vi "GUI_148_BeamPointingCams.vi"() -> ()   [LabVIEW 2013]
uses:
  Shared/GUI_Template/GUI_master/tcp_new_data_event.ctl
  Shared/GUI_Template/GUI_master/tcp new data cluster.ctl
  Control 2.ctl
  General GUIs/Device GUIs/GUI_Cameras/Controls/Crosshair type def.ctl
  <userlib>/_OpenG.lib/array/array.llb/Filter 1D Array with Scalar (String)__ogtk.vi
panel:
  in  "kHzMode":bool
  in  "DiodeMode":bool
  in  "Analysis::10":bool
  out "MeanCounts::10":dbl caption="updating?" min=0.0 max=999999999.0 format="%_4g"
  in  "Analysis::9":bool
  out "MeanCounts::9":dbl caption="updating?" min=0.0 max=999999999.0 format="%_4g"
  in  "Analysis::8":bool
  out "MeanCounts::8":dbl caption="updating?" min=0.0 max=999999999.0 format="%_4g"
  in  "Analysis::7":bool
  out "MeanCounts::7":dbl caption="updating?" min=0.0 max=999999999.0 format="%_4g"
  in  "Analysis::6":bool
  out "MeanCounts::6":dbl caption="updating?" min=0.0 max=999999999.0 format="%_4g"
  in  "Analysis::5":bool
  out "MeanCounts::5":dbl caption="updating?" min=0.0 max=999999999.0 format="%_4g"
  in  "Analysis::4":bool
  out "MeanCounts::4":dbl caption="updating?" min=0.0 max=999999999.0 format="%_4g"
  in  "Analysis::3":bool
  out "MeanCounts::3":dbl caption="updating?" min=0.0 max=999999999.0 format="%_4g"
  in  "Analysis::2":bool
  out "MeanCounts::2":dbl caption="updating?" min=0.0 max=999999999.0 format="%_4g"
  in  "Target.Y::10":dbl=45.0 caption="y" min=0.0 max=2000.0 format="%#_6f"
  in  "Target.X::10":dbl=47.0 caption="x" min=0.0 max=2000.0 format="%#_6f"
  in  "TargetSize.Y::10":dbl=45.0 caption="y" min=2.0 max=3000.0 format="%#_6f"
  in  "TargetSize.X::10":dbl=47.0 caption="x" min=2.0 max=3000.0 format="%#_6f"
  out "image::10":T1(plugin-control) caption="UC_BCaveIn"
  in  "GUIdevice 10":T2="UC_BCaveIn"
  in  "exposure::10":dbl=0.001 caption="exposure" min=10.0 max=1000000.0 format="%_4p"
  out "image::8":T1(plugin-control) caption="UC_Beamline_In"
  in  "GUIdevice 8":T2="UC_Beamline_In"
  in  "triggerdelay::10":dbl=0.001 caption="triggerdelay" min=10.0 max=1000000.0 format="%_4p"
  in  "triggerdelay::9":dbl=0.001 caption="triggerdelay" min=20.0 max=500000.0 format="%_4p"
  in  "triggerdelay::8":dbl=0.001 caption="triggerdelay" min=0.0 max=900000.0 format="%_4p"
  in  "trigger::10":bool caption="Trigger"
  in  "trigger::9":bool caption="Trigger"
  in  "trigger::8":bool caption="Trigger"
  in  "exposure::9":dbl=0.001 caption="exposure" min=0.0001 max=1.0 format="%_4p"
  in  "exposure::8":dbl=0.001 caption="exposure" min=0.0001 max=1.0 format="%_4p"
  in  "TargetSize.Y::9":dbl=45.0 caption="y" min=2.0 max=3000.0 format="%#_6f"
  in  "TargetSize.X::9":dbl=47.0 caption="x" min=2.0 max=3000.0 format="%#_6f"
  in  "TargetSize.Y::8":dbl=45.0 caption="y" min=2.0 max=3000.0 format="%#_6f"
  in  "TargetSize.X::8":dbl=47.0 caption="x" min=2.0 max=3000.0 format="%#_6f"
  in  "Target.Y::9":dbl=45.0 caption="y" min=0.0 max=2000.0 format="%#_6f"
  in  "Target.X::9":dbl=47.0 caption="x" min=0.0 max=2000.0 format="%#_6f"
  in  "Target.Y::8":dbl=45.0 caption="y" min=0.0 max=2000.0 format="%#_6f"
  in  "Target.X::8":dbl=47.0 caption="x" min=0.0 max=2000.0 format="%#_6f"
  out "image::9":T1(plugin-control) caption="UC_Beamline_Out"
  in  "GUIdevice 9":T2="UC_Beamline_Out"
  in  "Color Box":u32(colorbox)
  in  "TargetSize.Y::7":dbl=45.0 caption="y" min=2.0 max=3000.0 format="%#_6f"
  in  "TargetSize.X::7":dbl=47.0 caption="x" min=2.0 max=3000.0 format="%#_6f"
  in  "TargetSize.Y::6":dbl=45.0 caption="y" min=2.0 max=3000.0 format="%#_6f"
  in  "TargetSize.X::6":dbl=47.0 caption="x" min=2.0 max=3000.0 format="%#_6f"
  in  "TargetSize.Y::5":dbl=45.0 caption="y" min=2.0 max=3000.0 format="%#_6f"
  in  "TargetSize.X::5":dbl=47.0 caption="x" min=2.0 max=3000.0 format="%#_6f"
  in  "TargetSize.Y::4":dbl=45.0 caption="y" min=2.0 max=3000.0 format="%#_6f"
  in  "TargetSize.X::4":dbl=47.0 caption="x" min=2.0 max=3000.0 format="%#_6f"
  in  "TargetSize.Y::3":dbl=163.0 caption="y" min=2.0 max=3000.0 format="%#_6f"
  in  "TargetSize.X::3":dbl=152.0 caption="x" min=2.0 max=3000.0 format="%#_6f"
  in  "TargetSize.Y::2":dbl=74.0 caption="y" min=2.0 max=3000.0 format="%#_6f"
  in  "TargetSize.X::2":dbl=75.0 caption="x" min=2.0 max=3000.0 format="%#_6f"
  in  "active cams":string
  out "CCDs":string[](array[string])
  out "Cameras":T3
  in  "Target.Y::7":dbl=45.0 caption="y" min=0.0 max=2000.0 format="%#_6f"
  in  "Target.X::7":dbl=47.0 caption="x" min=0.0 max=2000.0 format="%#_6f"
  in  "Target.Y::6":dbl=45.0 caption="y" min=0.0 max=2000.0 format="%#_6f"
  in  "Target.X::6":dbl=47.0 caption="x" min=0.0 max=2000.0 format="%#_6f"
  in  "Target.Y::5":dbl=45.0 caption="y" min=0.0 max=2000.0 format="%#_6f"
  in  "Target.X::5":dbl=47.0 caption="x" min=0.0 max=2000.0 format="%#_6f"
  in  "Target.Y::4":dbl=45.0 caption="y" min=0.0 max=2000.0 format="%#_6f"
  in  "Target.X::4":dbl=47.0 caption="x" min=0.0 max=2000.0 format="%#_6f"
  in  "Target.Y::3":dbl=163.0 caption="y" min=0.0 max=2000.0 format="%#_6f"
  in  "Target.X::3":dbl=152.0 caption="x" min=0.0 max=2000.0 format="%#_6f"
  in  "Target.Y::2":dbl=74.0 caption="y" min=0.0 max=2000.0 format="%#_6f"
  in  "Target.X::2":dbl=75.0 caption="x" min=0.0 max=2000.0 format="%#_6f"
  out "error out":errorcluster
  out "image::7":T1(plugin-control) caption="UC_OAPin2"
  in  "triggerdelay::7":dbl=0.001 caption="triggerdelay" min=0.0 max=900000.0 format="%_4p"
  in  "triggerdelay::6":dbl=0.001 caption="triggerdelay" min=0.0 max=100000.0 format="%_4p"
  in  "triggerdelay::5":dbl=0.001 caption="triggerdelay" min=0.0 max=100000.0 format="%_4p"
  in  "triggerdelay::4":dbl=0.001 caption="triggerdelay" min=0.01 max=999000.0 format="%_4p"
  in  "triggerdelay::3":dbl=0.001 caption="triggerdelay" min=0.0 max=100000.0 format="%_4p"
  in  "triggerdelay::2":dbl=0.001 caption="triggerdelay" min=0.0 max=50000.0 format="%_4p"
  in  "trigger::7":bool caption="Trigger"
  in  "exposure::7":dbl=0.001 caption="exposure" min=0.0001 max=1.0 format="%_4p"
  in  "GUIdevice 7":string="UC_OAPin2"
  in  "trigger::6":bool caption="Trigger"
  in  "exposure::6":dbl=0.001 caption="exposure" min=0.0001 max=1.0 format="%_4p"
  out "image::6":T1(plugin-control) caption="UC_OAPin1"
  in  "GUIdevice 6":string="UC_OAPin1"
  in  "trigger::5":bool caption="Trigger"
  in  "exposure::5":dbl=0.001 caption="exposure" min=2e-05 max=1.0 format="%_4p"
  out "image::5":T1(plugin-control) caption="UC_CompIn"
  in  "GUIdevice 5":string="UC_CompIn"
  in  "trigger::4":bool caption="Trigger"
  in  "exposure::4":dbl=0.001 caption="exposure" min=50.0 max=500000.0 format="%_4p"
  out "image::4":T1(plugin-control) caption="UC_TubeIn"
  in  "GUIdevice 4":string="UC_TubeIn"
  in  "trigger::3":bool caption="Trigger"
  in  "exposure::3":dbl=0.001 caption="exposure" min=3e-05 max=1.0 format="%_4p"
  out "image::3":T1(plugin-control) caption="UC_ExpanderIn2"
  in  "GUIdevice 3":string="UC_ExpanderIn2"
  in  "trigger::2":bool caption="Trigger"
  in  "exposure::2":dbl=0.001 caption="exposure" min=1e-06 max=1.0 format="%_4p"
  out "image::2":T1(plugin-control) caption="UC_ExpanderIn1_Pulsed"
  in  "GUIdevice 2":string="UC_ExpanderIn1_Pulsed"
  out "tcp data event":T4
  in  "Refresh Button":bool caption="Update Crosshairs"
  in  "Select device":string(combo)="FrogHPD"
  in  "stop":bool
  in  "GUIdevice 1":string="HPD_CCD"
  # "XHair location"
  # "XHair size"
  # "XHair size"
  # "XHair location"
  # "XHair size"
  # "XHair location"
  # "XHair size"
  # "XHair location"
  # "XHair location"
  # "XHair size"
  # "XHair location"
  # "XHair size"
  # "XHair location"
  # "XHair size"
  # "XHair size"
  # "XHair location"
  # "XHair size"
  # "XHair location"
  # "XHair size"
  # "XHair location"
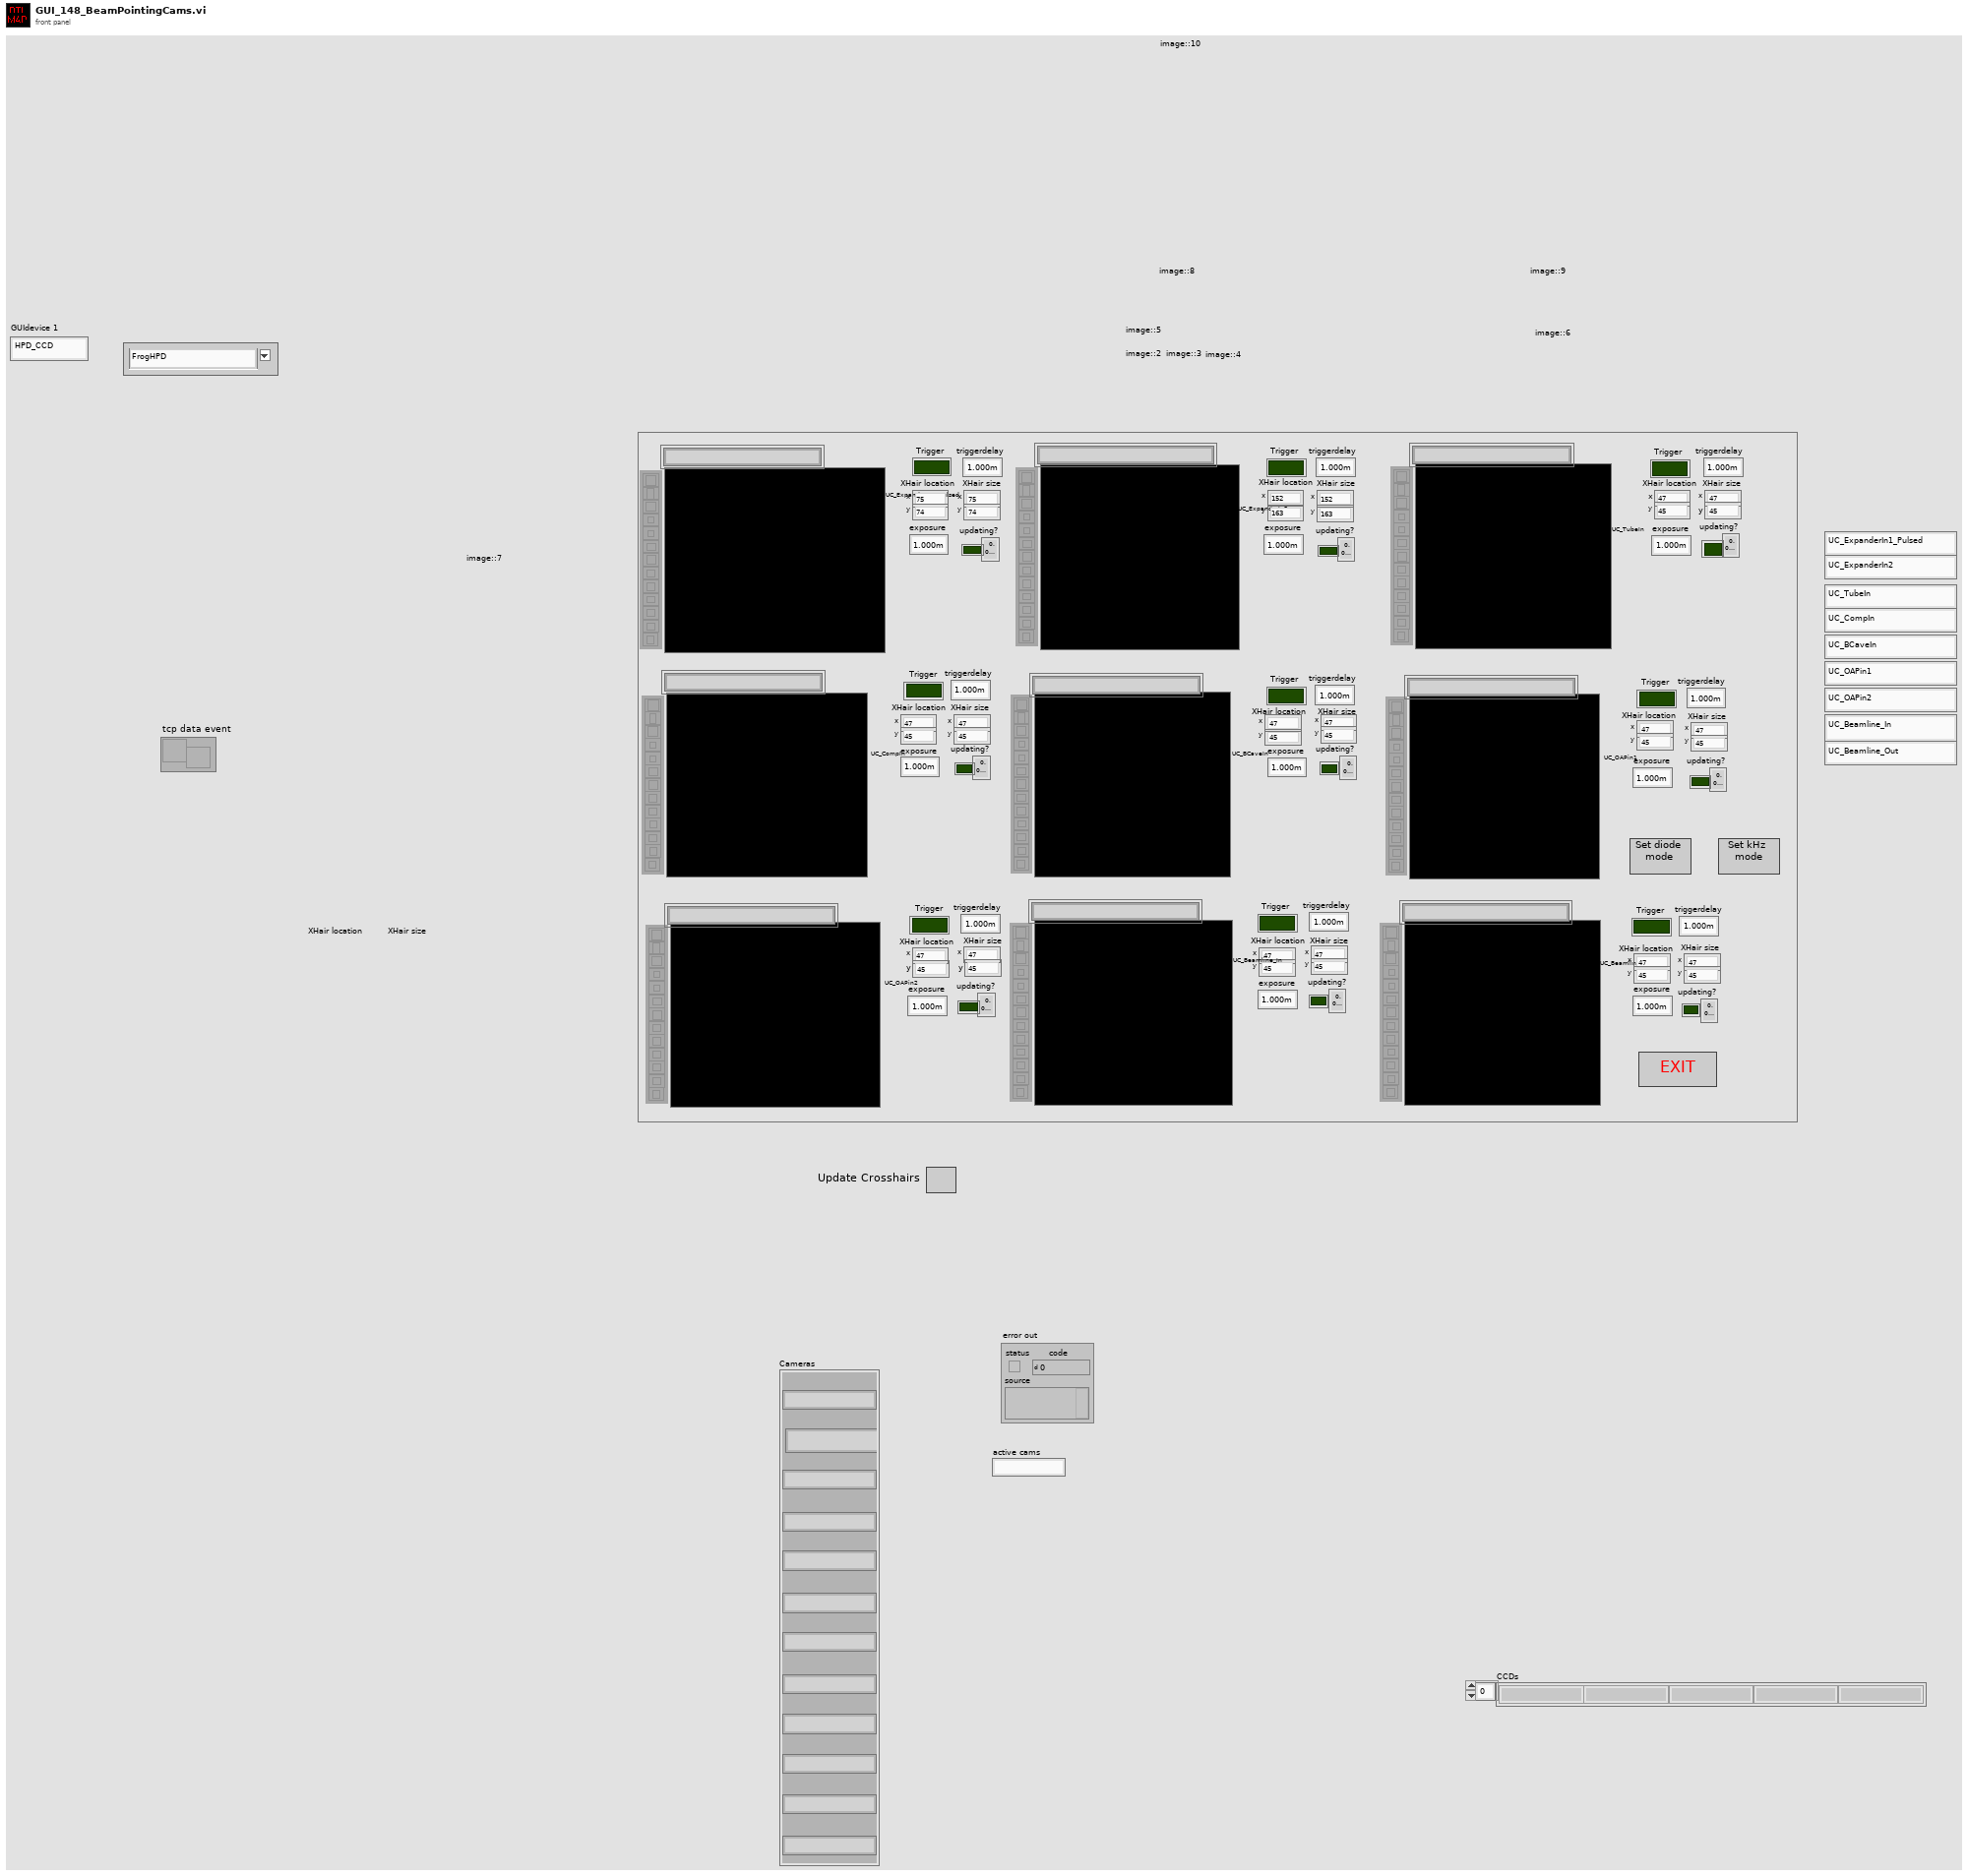
[diagram p1: front panel]
types:
  T1 = typedef "IMAQ Image.ctl" = refnum<image>
  T2 = typedef "Control 2.ctl" = string
  T3 = cluster{"[0]":string, "[1]":string, "[2]":string, "[3]":string, "[4]":string, "[5]":string, "[6]":string, "[7]":string, "[8]":string, "[8] 2":string, "[8] 3":string, "[8] 4":string}
  T4 = typedef "tcp_new_data_event.ctl" = refnum<user-event>
  T5 = typedef "Image Type" = u32
  T6 = cluster{"Target.X::8":refnum<vi>, "Target.Y::8":refnum<vi>}
  T7 = cluster{"Target.X::9":refnum<vi>, "Target.Y::9":refnum<vi>}
  T8 = cluster{"Target.X::10":refnum<vi>, "Target.Y::10":refnum<vi>}
  T9 = cluster{"TargetSize.X::2":refnum<vi>, "TargetSize.Y::2":refnum<vi>}
  T10 = cluster{"TargetSize.X::3":refnum<vi>, "TargetSize.Y::3":refnum<vi>}
  T11 = cluster{"TargetSize.X::4":refnum<vi>, "TargetSize.Y::4":refnum<vi>}
  T12 = cluster{"TargetSize.X::5":refnum<vi>, "TargetSize.Y::5":refnum<vi>}
  T13 = cluster{"TargetSize.X::6":refnum<vi>, "TargetSize.Y::6":refnum<vi>}
  T14 = cluster{"TargetSize.X::7":refnum<vi>, "TargetSize.Y::7":refnum<vi>}
  T15 = cluster{"Target.X::2":refnum<vi>, "Target.Y::2":refnum<vi>}
  T16 = cluster{"Target.X::3":refnum<vi>, "Target.Y::3":refnum<vi>}
  T17 = cluster{"Target.X::4":refnum<vi>, "Target.Y::4":refnum<vi>}
  T18 = cluster{"Target.X::5":refnum<vi>, "Target.Y::5":refnum<vi>}
  T19 = cluster{"Target.X::6":refnum<vi>, "Target.Y::6":refnum<vi>}
  T20 = cluster{"Target.X::7":refnum<vi>, "Target.Y::7":refnum<vi>}
  T21 = cluster{"TargetSize.Y::8":refnum<vi>, "TargetSize.X::8":refnum<vi>}
  T22 = cluster{"TargetSize.Y::9":refnum<vi>, "TargetSize.X::9":refnum<vi>}
  T23 = cluster{"TargetSize.Y::10":refnum<vi>, "TargetSize.X::10":refnum<vi>}
  T24 = cluster{"[0]":T2, "[1]":T2, "[2]":T2, "[3]":T2, "[4]":T2, "[5]":T2, "[6]":T2, "[7]":T2, "[8]":T2, "[9]":T2, "[10]":T2, "[11]":T2}
  T25 = cluster{"TargetSize.Y::10":refnum<vi>, "TargetSize.X::10":refnum<vi>}[]
  T26 = cluster{"Target.X::10":refnum<vi>, "Target.Y::10":refnum<vi>}[]
  T27 = typedef "Crosshair type def.ctl" = cluster{"Draw":bool, "Target":cluster{"x":dbl, "y":dbl}, "Size":cluster{"x":dbl, "y":dbl}, "Angle":dbl, "Color":u32, "Thickness":u8, "CrosshairLabel":string}
  T28 = cluster{"Left":i32, "Top":i32, "Right":i32, "Bottom":i32}
  T29 = enum32{"invalid app kind", "Development System", "Run Time System", "Student Edition", "Embedded LabVIEW", "Evaluation", "Custom"}
  T30 = typedef "tcp new data cluster.ctl" = cluster{"EventEnum":enum16{"new data", "connection status update"}, "Device name":string}
  T31 = enum32{"Invalid", "Standard", "Closed", "Hidden", "Minimized", "Maximized"}
  T32 = cluster{"Core":cluster{"Current VI Reference":refnum<vi>, "Close Panel on Exit?":bool}, "DiodeMode":bool, "active cams":string, "SuperGUI":cluster{"STOP queue":refnum<queue>, "SuperGUI ref":refnum<vi>}, "kHzMode":bool}
  T33 = cluster{"STOP queue":refnum<queue>, "SuperGUI ref":refnum<vi>}
  T34 = cluster{"Current VI Reference":refnum<vi>, "Close Panel on Exit?":bool}
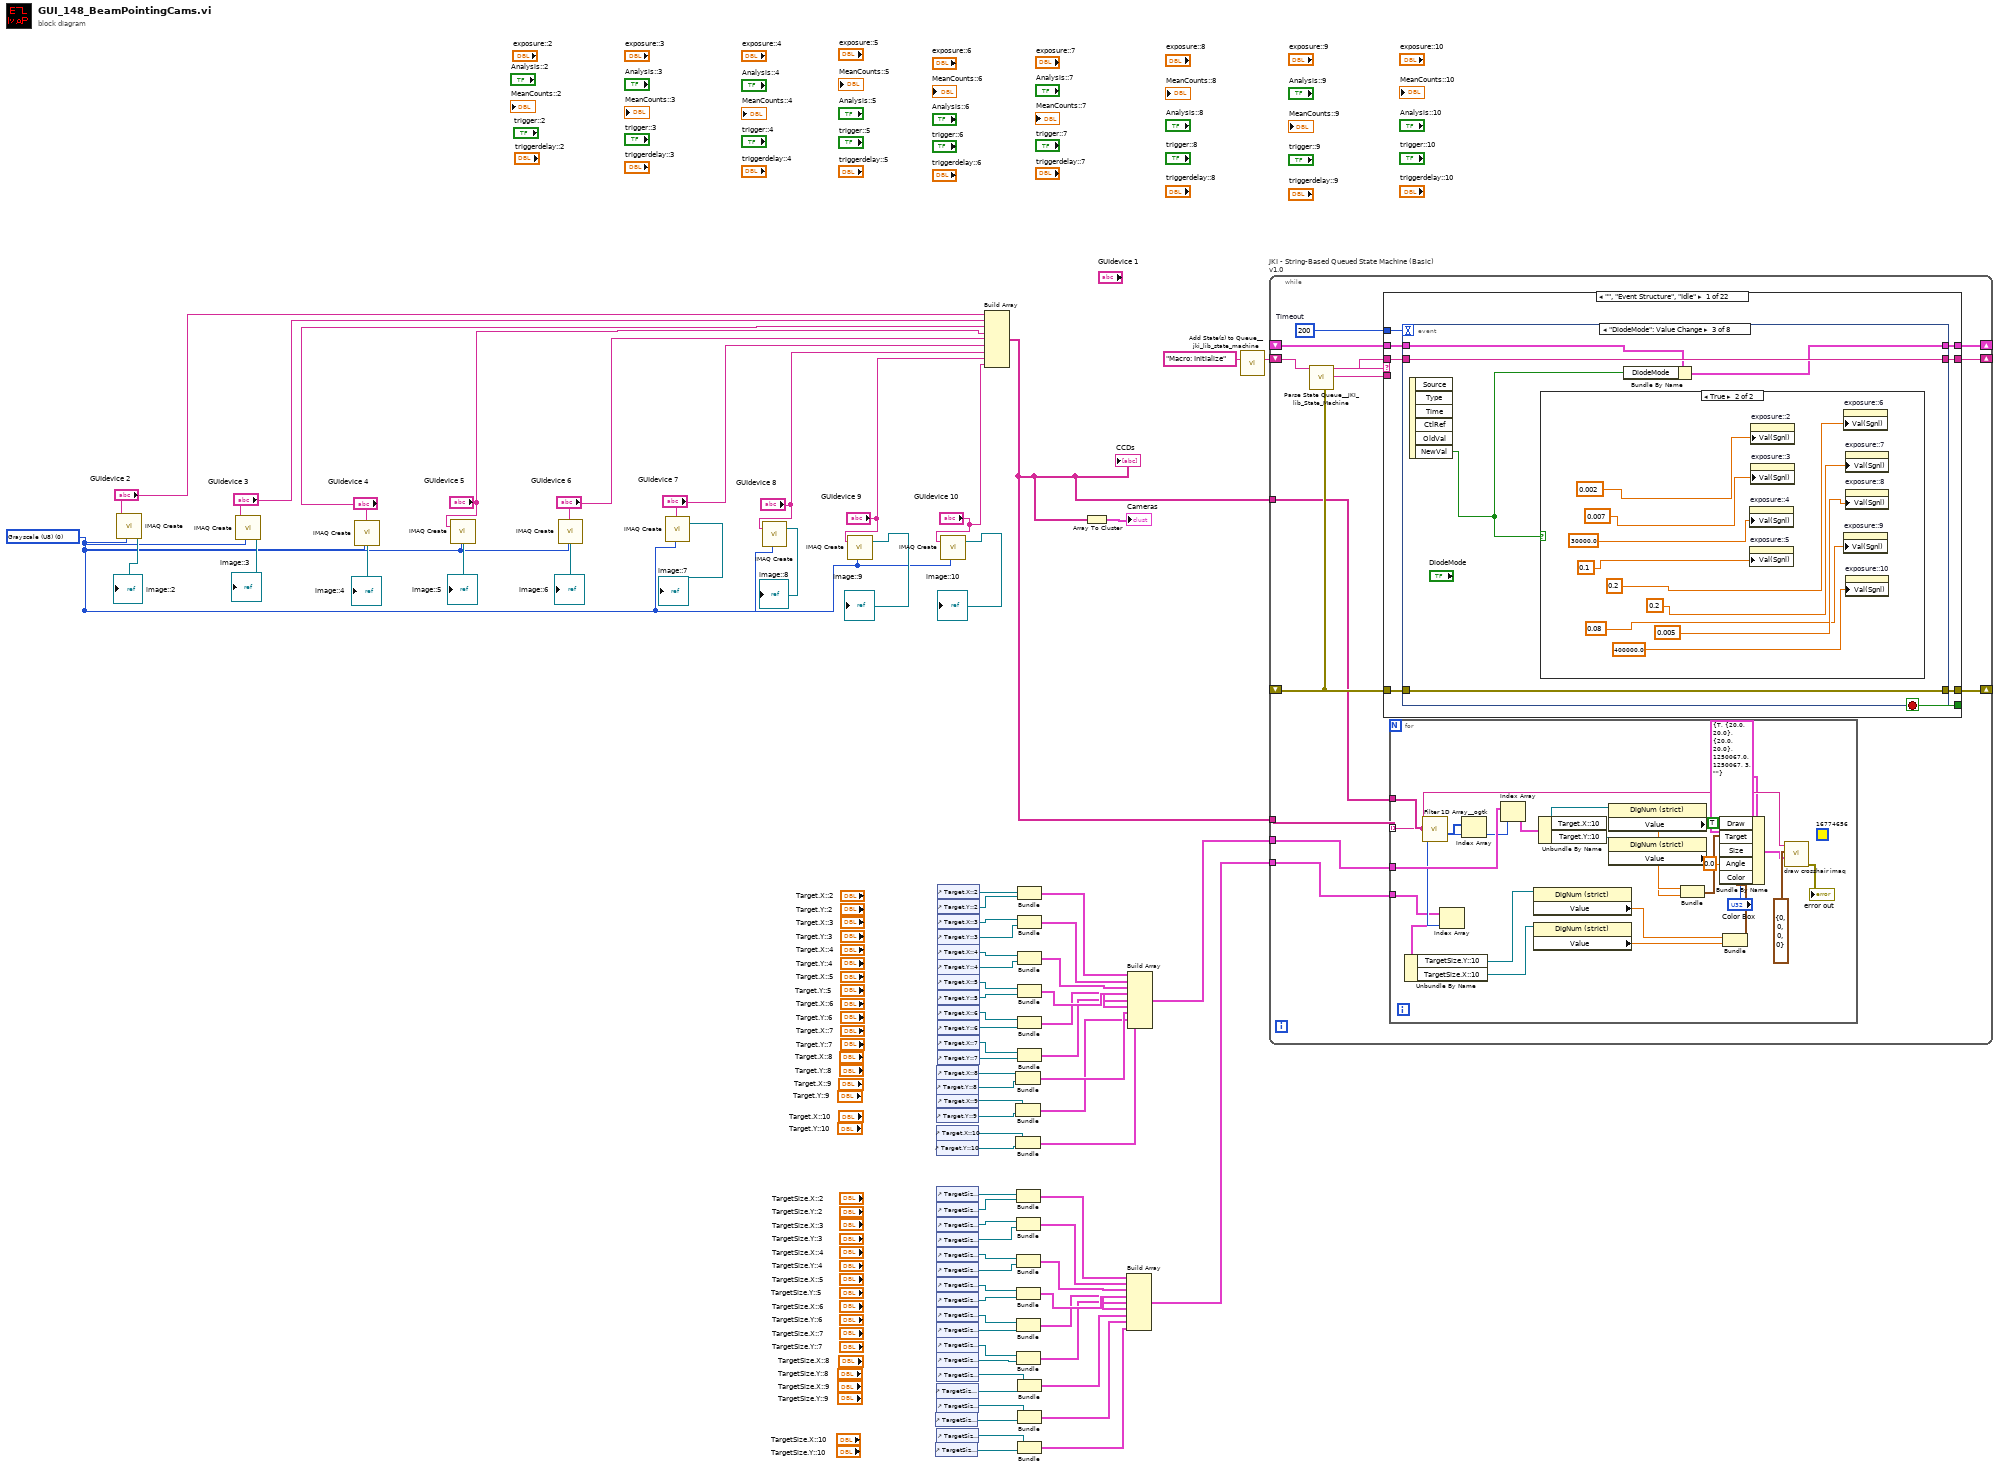
[diagram p0: block diagram]
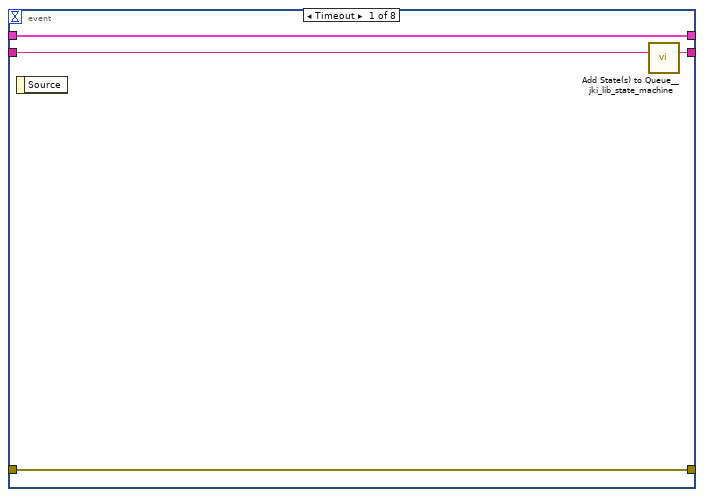
[diagram p2: hidden frame]
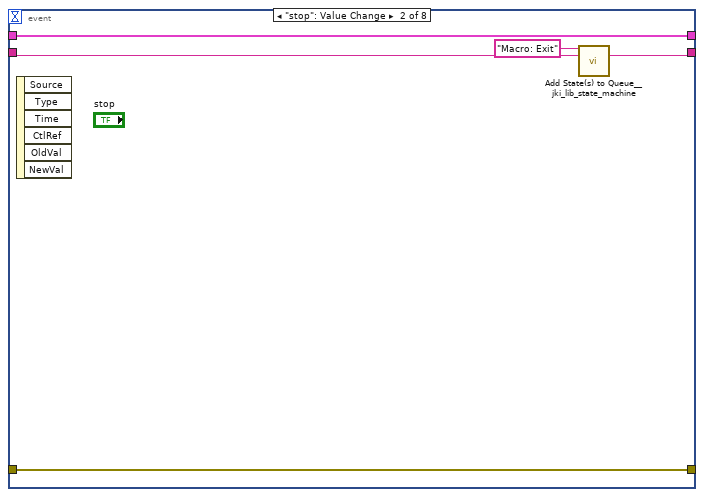
[diagram p3: hidden frame]
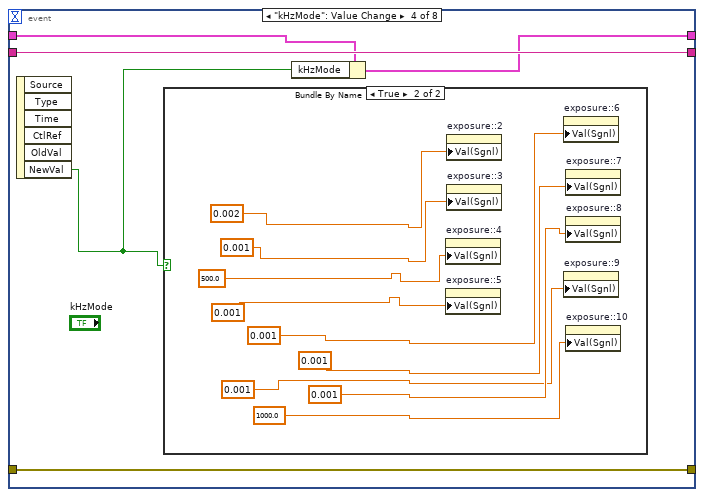
[diagram p5: hidden frame]
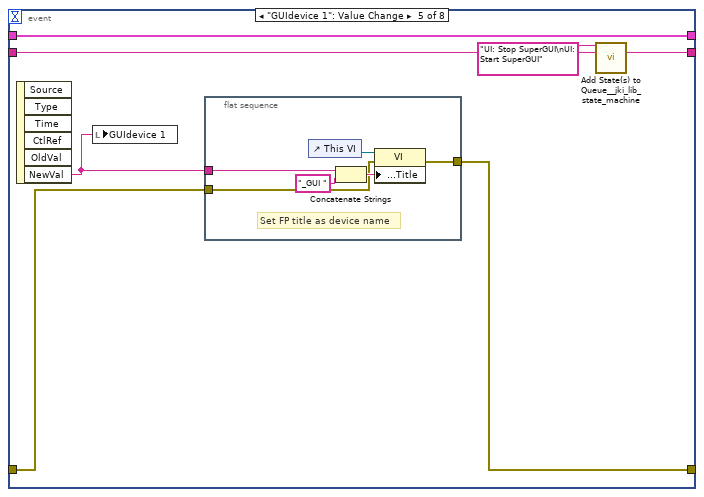
[diagram p7: hidden frame]
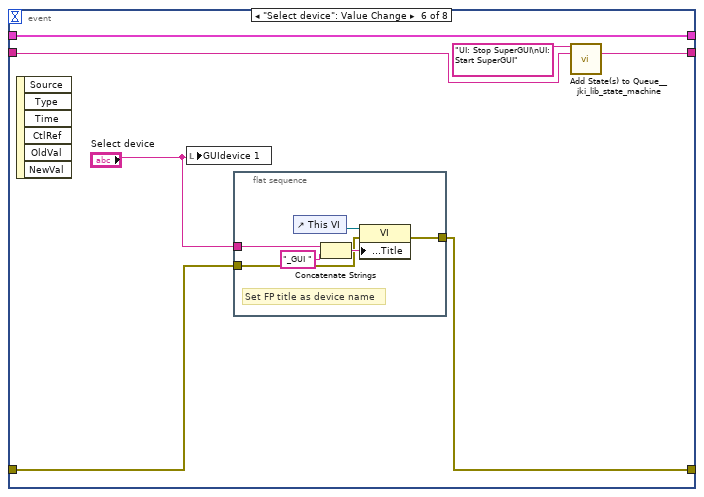
[diagram p8: hidden frame]
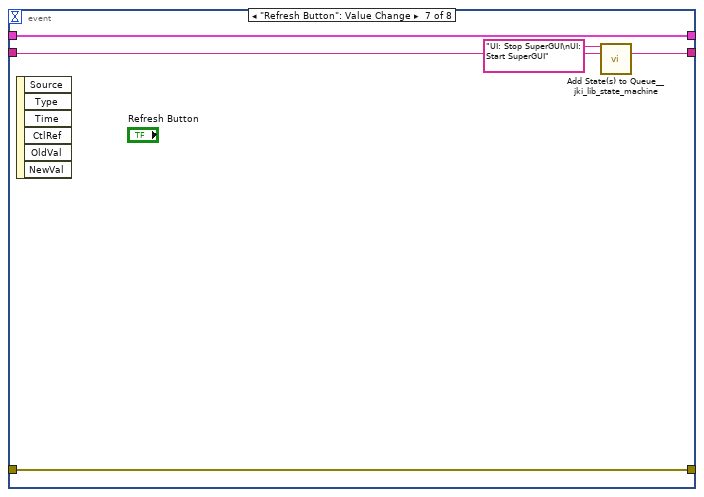
[diagram p9: hidden frame]
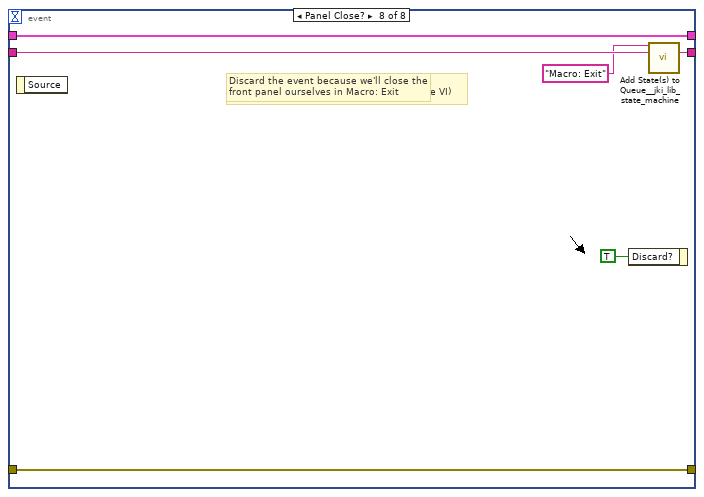
[diagram p10: hidden frame]
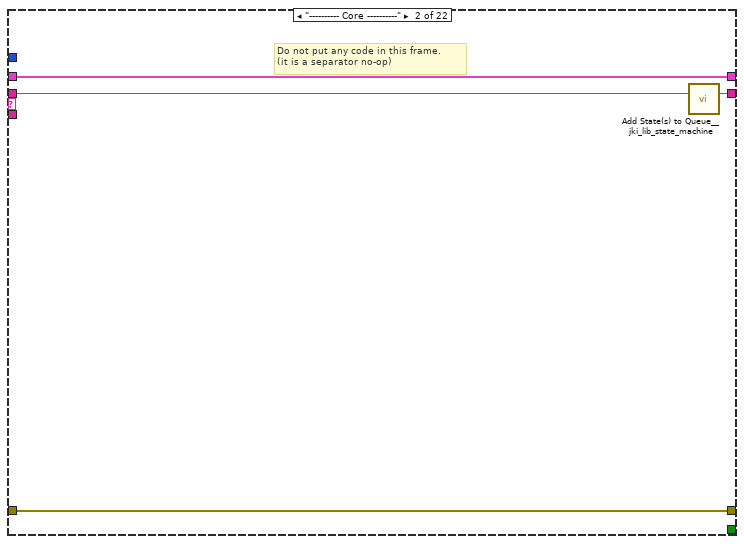
[diagram p11: hidden frame]
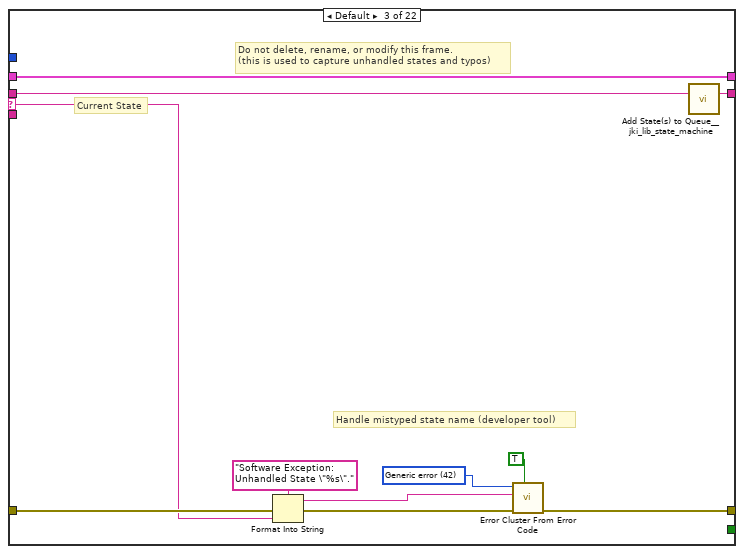
[diagram p12: hidden frame]
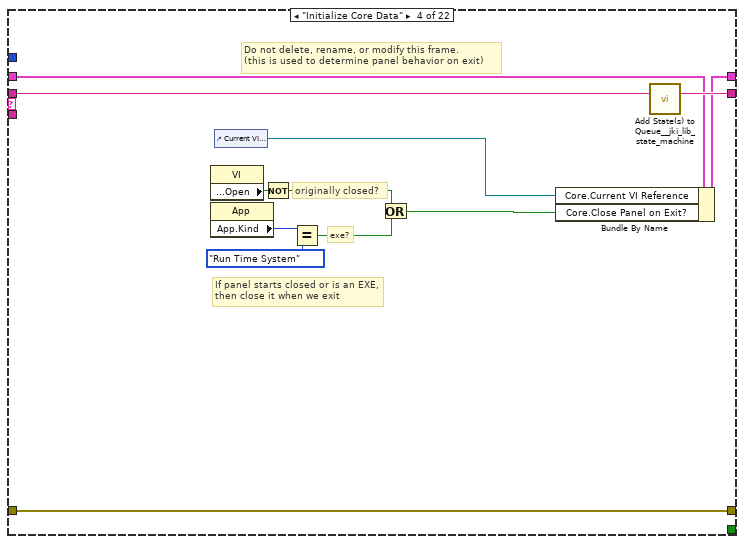
[diagram p13: hidden frame]
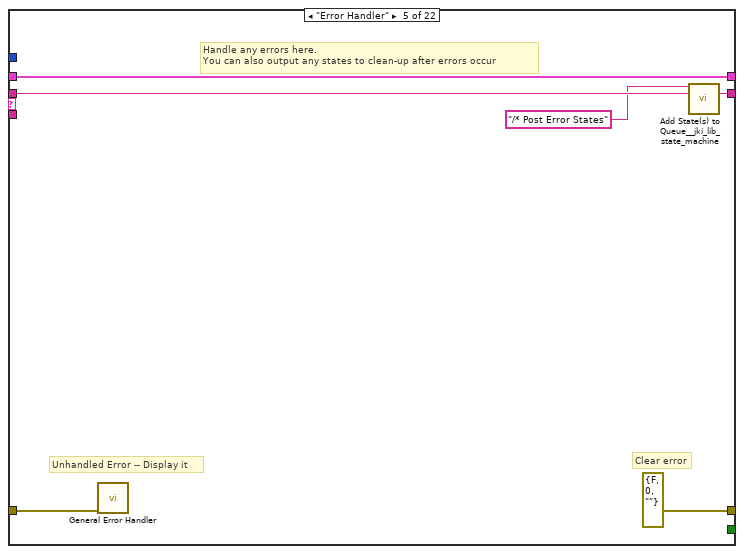
[diagram p14: hidden frame]
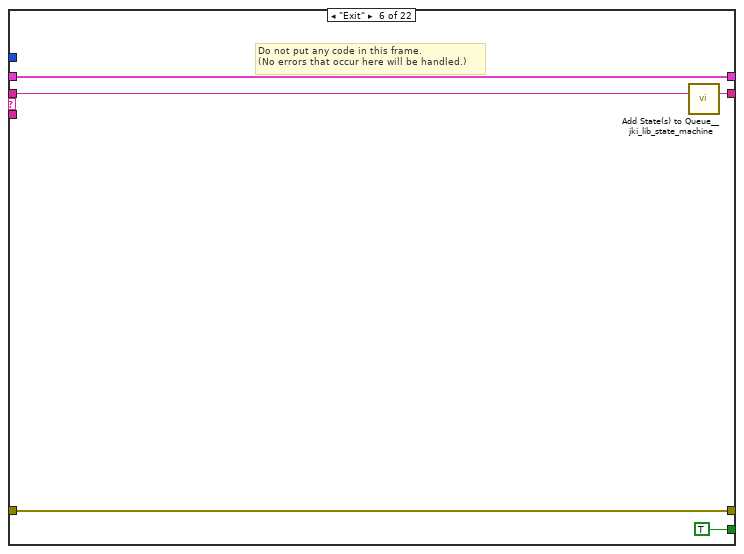
[diagram p15: hidden frame]
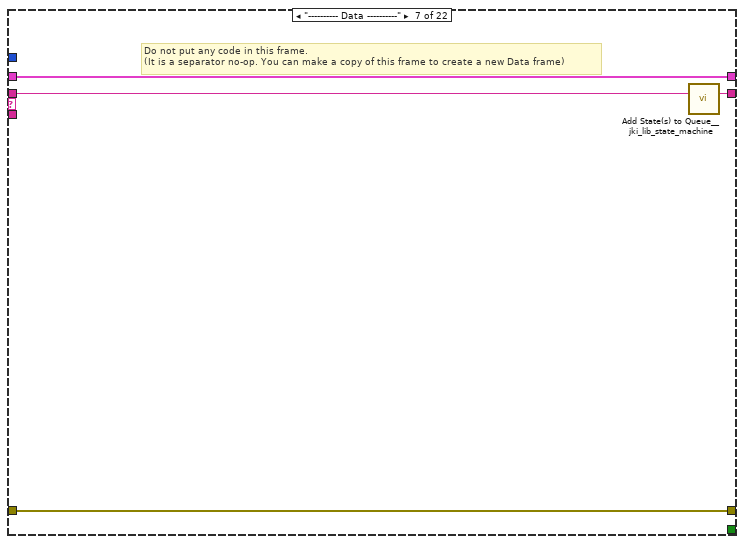
[diagram p16: hidden frame]
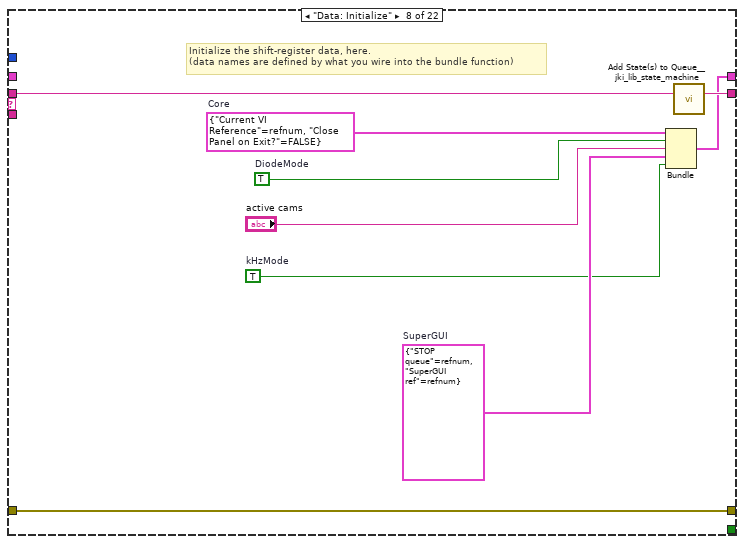
[diagram p17: hidden frame]
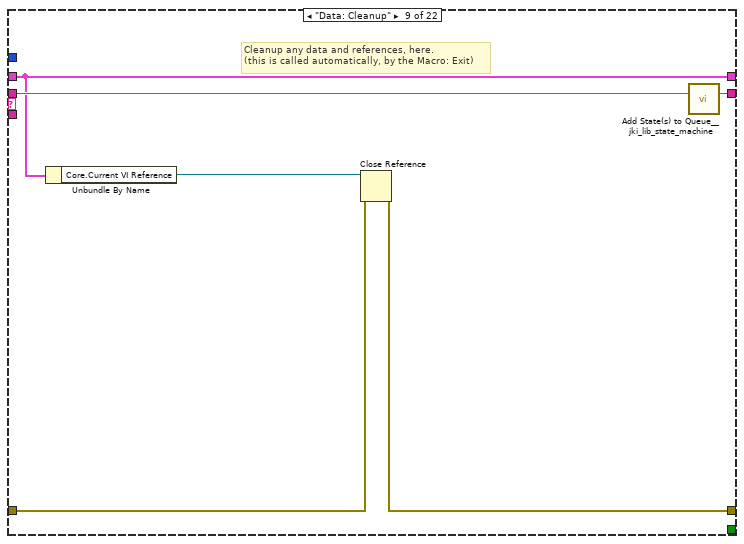
[diagram p18: hidden frame]
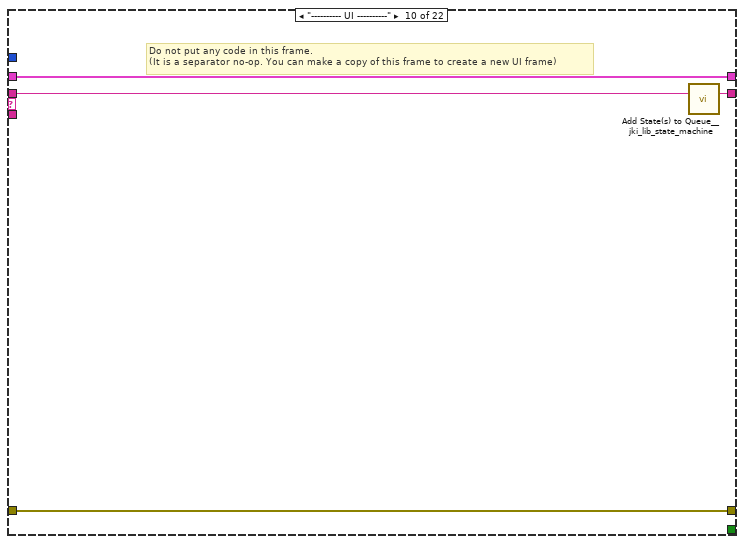
[diagram p19: hidden frame]
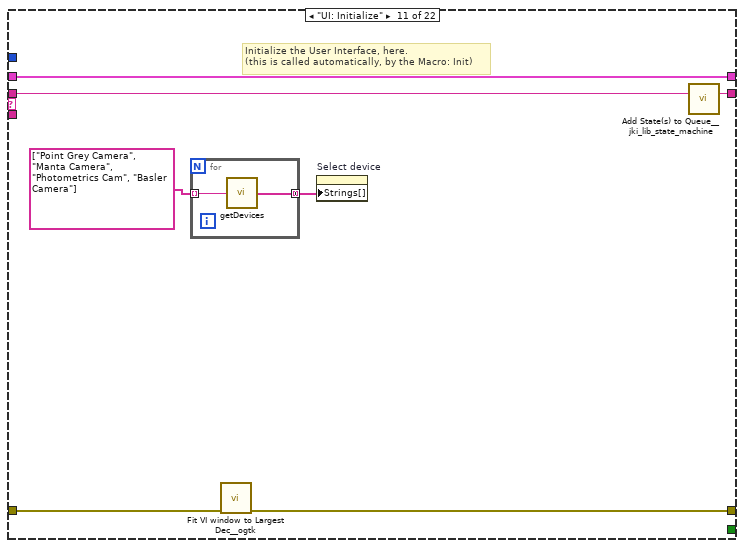
[diagram p20: hidden frame]
diagram:
  w8 = T5 0 items=["Grayscale (U8)", "Grayscale (I16)", "Grayscale (SGL)", "Complex (CSG)", "RGB (U32)", "HSL (U32)", "RGB (U64)", "Grayscale (U16)"] ("Image Type")
  n1 = call "IMAQ Create"("Image Name"="GUIdevice 2", "Image Type"=w8) -> ("New Image"=→"image::2":T1)  [unwired: 3 in, 1 out]
  n2 = call "IMAQ Create"("Image Name"="GUIdevice 3", "Image Type"=w8) -> ("New Image"=→"image::3":T1)  [unwired: 3 in, 1 out]
  n3 = call "IMAQ Create"("Image Name"="GUIdevice 4", "Image Type"=w8) -> ("New Image"=→"image::4":T1)  [unwired: 3 in, 1 out]
  n4 = call "IMAQ Create"("Image Name"="GUIdevice 5", "Image Type"=w8) -> ("New Image"=→"image::5":T1)  [unwired: 3 in, 1 out]
  n5 = call "IMAQ Create"("Image Name"="GUIdevice 6", "Image Type"=w8) -> ("New Image"=→"image::6":T1)  [unwired: 3 in, 1 out]
  n6 = call "IMAQ Create"("Image Name"="GUIdevice 7", "Image Type"=w8) -> ("New Image"=→"image::7":T1)  [unwired: 3 in, 1 out]
  n7 = call "IMAQ Create"("Image Name"="GUIdevice 8", "Image Type"=w8) -> ("New Image"=→"image::8":T1)  [unwired: 3 in, 1 out]
  n8 = call "IMAQ Create"("Image Name"="GUIdevice 9", "Image Type"=w8) -> ("New Image"=→"image::9":T1)  [unwired: 3 in, 1 out]
  n9 = control-ref of="TargetSize.X::9"() -> (w13:refnum<vi>)
  n10 = control-ref of="TargetSize.X::10"() -> (w5:refnum<vi>)
  n11 = control-ref of="Target.Y::8"() -> (w23:refnum<vi>)
  n12 = control-ref of="Target.Y::9"() -> (w20:refnum<vi>)
  n13 = control-ref of="Target.Y::10"() -> (w2:refnum<vi>)
  n14 = control-ref of="TargetSize.X::8"() -> (w15:refnum<vi>)
  n15 = control-ref of="Target.X::8"() -> (w24:refnum<vi>)
  n16 = control-ref of="Target.X::9"() -> (w21:refnum<vi>)
  n17 = control-ref of="Target.X::10"() -> (w3:refnum<vi>)
  n18 = control-ref of="TargetSize.X::2"() -> (w44:refnum<vi>)
  n19 = control-ref of="TargetSize.Y::2"() -> (w43:refnum<vi>)
  n20 = control-ref of="TargetSize.X::3"() -> (w42:refnum<vi>)
  n21 = control-ref of="TargetSize.Y::3"() -> (w41:refnum<vi>)
  n22 = control-ref of="TargetSize.X::4"() -> (w40:refnum<vi>)
  n23 = control-ref of="TargetSize.Y::4"() -> (w39:refnum<vi>)
  n24 = control-ref of="TargetSize.X::5"() -> (w38:refnum<vi>)
  n25 = control-ref of="TargetSize.Y::5"() -> (w37:refnum<vi>)
  n26 = control-ref of="TargetSize.X::6"() -> (w36:refnum<vi>)
  n27 = control-ref of="TargetSize.Y::6"() -> (w35:refnum<vi>)
  n28 = control-ref of="TargetSize.X::7"() -> (w34:refnum<vi>)
  n29 = control-ref of="TargetSize.Y::7"() -> (w33:refnum<vi>)
  n30 = control-ref of="TargetSize.Y::8"() -> (w16:refnum<vi>)
  n31 = control-ref of="TargetSize.Y::9"() -> (w14:refnum<vi>)
  n32 = control-ref of="TargetSize.Y::10"() -> (w6:refnum<vi>)
  n33 = control-ref of="Target.X::2"() -> (w71:refnum<vi>)
  n34 = control-ref of="Target.Y::2"() -> (w70:refnum<vi>)
  n35 = control-ref of="Target.X::3"() -> (w69:refnum<vi>)
  n36 = control-ref of="Target.Y::3"() -> (w68:refnum<vi>)
  n37 = control-ref of="Target.X::4"() -> (w67:refnum<vi>)
  n38 = control-ref of="Target.Y::4"() -> (w66:refnum<vi>)
  n39 = control-ref of="Target.X::5"() -> (w65:refnum<vi>)
  n40 = control-ref of="Target.Y::5"() -> (w64:refnum<vi>)
  n41 = control-ref of="Target.X::6"() -> (w63:refnum<vi>)
  n42 = control-ref of="Target.Y::6"() -> (w62:refnum<vi>)
  n43 = control-ref of="Target.X::7"() -> (w61:refnum<vi>)
  n44 = control-ref of="Target.Y::7"() -> (w60:refnum<vi>)
  n45 = call "IMAQ Create"("Image Name"="GUIdevice 10", "Image Type"=w8) -> ("New Image"=→"image::10":T1)  [unwired: 3 in, 1 out]
  n46 = Build Array("GUIdevice 2", "GUIdevice 3", "GUIdevice 4", "GUIdevice 5", "GUIdevice 6", "GUIdevice 7", "GUIdevice 8", "GUIdevice 9", "GUIdevice 10") -> (w45:T2[])
  "CCDs" <- w45
  n47 = Bundle("Target.X::8"=w24, "Target.Y::8"=w23) -> (w22:T6)  [unwired: 1 in]
  n48 = Bundle("Target.X::9"=w21, "Target.Y::9"=w20) -> (w19:T7)  [unwired: 1 in]
  n49 = Bundle("Target.X::10"=w3, "Target.Y::10"=w2) -> (w1:T8)  [unwired: 1 in]
  n50 = Bundle("TargetSize.X::2"=w44, "TargetSize.Y::2"=w43) -> (w32:T9)  [unwired: 1 in]
  n51 = Bundle("TargetSize.X::3"=w42, "TargetSize.Y::3"=w41) -> (w31:T10)  [unwired: 1 in]
  n52 = Bundle("TargetSize.X::4"=w40, "TargetSize.Y::4"=w39) -> (w27:T11)  [unwired: 1 in]
  n53 = Bundle("TargetSize.X::5"=w38, "TargetSize.Y::5"=w37) -> (w30:T12)  [unwired: 1 in]
  n54 = Bundle("TargetSize.X::6"=w36, "TargetSize.Y::6"=w35) -> (w29:T13)  [unwired: 1 in]
  n55 = Bundle("TargetSize.X::7"=w34, "TargetSize.Y::7"=w33) -> (w28:T14)  [unwired: 1 in]
  n56 = Bundle("Target.X::2"=w71, "Target.Y::2"=w70) -> (w59:T15)  [unwired: 1 in]
  n57 = Bundle("Target.X::3"=w69, "Target.Y::3"=w68) -> (w58:T16)  [unwired: 1 in]
  n58 = Bundle("Target.X::4"=w67, "Target.Y::4"=w66) -> (w54:T17)  [unwired: 1 in]
  n59 = Bundle("Target.X::5"=w65, "Target.Y::5"=w64) -> (w57:T18)  [unwired: 1 in]
  n60 = Bundle("Target.X::6"=w63, "Target.Y::6"=w62) -> (w56:T19)  [unwired: 1 in]
  n61 = Bundle("Target.X::7"=w61, "Target.Y::7"=w60) -> (w55:T20)  [unwired: 1 in]
  n62 = Bundle("TargetSize.Y::8"=w16, "TargetSize.X::8"=w15) -> (w18:T21)  [unwired: 1 in]
  n63 = Bundle("TargetSize.Y::9"=w14, "TargetSize.X::9"=w13) -> (w17:T22)  [unwired: 1 in]
  n64 = Bundle("TargetSize.Y::10"=w6, "TargetSize.X::10"=w5) -> (w4:T23)  [unwired: 1 in]
  n65 = Array To Cluster(array=w45) -> (cluster=→"Cameras":T24)
  n66 = Build Array(w32, w31, w27, w30, w29, w28, w18, w17, w4) -> (w26:T25)
  n67 = Build Array(w59, w58, w54, w57, w56, w55, w22, w19, w1) -> (w53:T26)
  n68 = call <vilib>:"Add State(s) to Queue__jki_lib_state_machine.vi"("State(s) in (\"\")"="Macro: Initialize") -> ("States Out"=w79:string)  [unwired: 14 in]
  n69 = while "JKI - String-Based Queued State Machine (Basic) v1.0" {
    shift-right: [w87] -> _
    shift-left: _ -> [w82]
    shift-right: [w90] -> _
    shift-left: _ -> [w85]
    shift-right: [w89] -> _
    shift-left: w79 -> [w91]
    tunnel: w53 -> [w84]
    tunnel: w45 -> [w83]
    tunnel: w45 -> [w81]
    tunnel: w26 -> [w80]
    stop <- w88 stop-if-true
    w86 = 200  # Timeout
    n70 = call <vilib>:"Parse State Queue__JKI_lib_State_Machine.vi"("State Queue"=w91, "Error In (no error)"=w85) -> ("Remaining States"=w93:string, "Current State"=w94:string, "Arguments"=w92:string)  [unwired: 11 in]
    n71 = case shown="\"\", \"Event Structure\", \"Idle\"" w94 {
      selector: w94 -> [_ _ w205 _ _ _ _ _ _ _ _ _ _ _ _ _ _ _ _ _ _ _]
      tunnel: w93 -> [w126 w204 w209 w227 w233 w238 w242 w251 w257 w261 w268 w276 w311 w319 w325 w336 w362 w367 w377 w381 w385 w389]
      tunnel: w92 -> [_ _ _ _ _ _ _ _ _ _ _ _ _ _ w320 w330 _ _ _ _ _ _]
      tunnel: w82 -> [w124 w201 w207 w218 w230 w236 w239 _ w252 w258 w266 w274 w302 w314 w323 w332 w359 w364 w374 w378 w382 w386]
      tunnel: [w123 w202 w211 w224 errorcluster {"status"=FALSE, "code"=0, "source"=""} ("error out") w235 w240 w248 w253 w259 w264 w271 w295 w312 w321 w333 w360 w365 w375 w379 w383 w387] -> w90
      tunnel: w85 -> [w122 w202 w210 w224 w229 w235 w240 w248 w254 w259 w265 w272 w296 w313 w322 w334 w360 w365 w375 w379 w383 w387]
      tunnel: [w125 w203 w208 w226 w232 w237 w241 w250 w256 w260 w267 w275 w310 w318 w324 w335 w361 w366 w376 w380 w384 w388] -> w89
      tunnel: [_ _ _ _ _ TRUE _ _ _ _ _ _ _ _ _ _ _ _ _ _ _ _] -> w88
      tunnel: [w121 w201 w207 w225 w230 w236 w239 w249 w252 w258 w266 w274 w301 w314 w323 w332 w359 w364 w374 w378 w382 w386] -> w87
      tunnel: w86 -> [w120 _ _ _ _ _ _ _ _ _ _ _ _ _ _ _ _ _ _ _ _ _]
      frame "", "Event Structure", "Idle" {
        n72 = event shown="[2] \"DiodeMode\": Value Change" {
          selector: _ -> [_ _ _ _ _ _ _ _]
          dyn-events: _ -> [_ _ _ _ _ _ _ _]
          timeout: w120 -> [_ _ _ _ _ _ _ _]
          tunnel: w126 -> [w130 w133 w139 w153 w167 w179 w192 w200]
          tunnel: [w129 w132 w139 w153 w166 w178 w191 w199] -> w125
          tunnel: w124 -> [w127 w135 w138 w152 w170 w183 w194 w197]
          tunnel: [w128 w134 w140 w154 w168 w181 w193 w198] -> w123
          tunnel: w122 -> [w128 w134 w140 w154 w169 w182 w193 w198]
          tunnel: [w127 w135 w137 w151 w170 w183 w194 w197] -> w121
          event Timeout {
            n73 = event-data() -> ()  [unwired: 1 in, 1 out]
            n74 = call <vilib>:"Add State(s) to Queue__jki_lib_state_machine.vi"("State(s) in (\"\")"=w130) -> ("States Out"=w129:string)  [unwired: 14 in]
          }
          event "stop": Value Change {
            n75 = event-data() -> ()  [unwired: 1 in, 6 out]
            n76 = call <vilib>:"Add State(s) to Queue__jki_lib_state_machine.vi"("State(s) in Front (\"\")"="Macro: Exit", "State(s) in (\"\")"=w133) -> ("States Out"=w132:string)  [unwired: 13 in]
          }
          event "DiodeMode": Value Change {
            n77 = event-data() -> ("NewVal"=w136:bool)  [unwired: 1 in, 5 out]
            n78 = case shown="True" w136 {
              frame False {
              }
              frame True {
                n79 = property on="exposure::4" class="DigNum (strict)"("Val(Sgnl)"=30000.0) -> ()  [unwired: 2 in, 2 out]
                n80 = property on="exposure::5" class="DigNum (strict)"("Val(Sgnl)"=0.1) -> ()  [unwired: 2 in, 2 out]
                n81 = property on="exposure::2" class="DigNum (strict)"("Val(Sgnl)"=0.002) -> ()  [unwired: 2 in, 2 out]
                n82 = property on="exposure::3" class="DigNum (strict)"("Val(Sgnl)"=0.007) -> ()  [unwired: 2 in, 2 out]
                n83 = property on="exposure::6" class="DigNum (strict)"("Val(Sgnl)"=0.2) -> ()  [unwired: 2 in, 2 out]
                n84 = property on="exposure::9" class="DigNum (strict)"("Val(Sgnl)"=0.08) -> ()  [unwired: 2 in, 2 out]
                n85 = property on="exposure::7" class="DigNum (strict)"("Val(Sgnl)"=0.2) -> ()  [unwired: 2 in, 2 out]
                n86 = property on="exposure::8" class="DigNum (strict)"("Val(Sgnl)"=0.005) -> ()  [unwired: 2 in, 2 out]
                n87 = property on="exposure::10" class="DigNum (strict)"("Val(Sgnl)"=400000.0) -> ()  [unwired: 2 in, 2 out]
              }
            }
            n88 = Bundle By Name(cluster=w138, "DiodeMode"=w136) -> (w137:T32)
          }
          event "kHzMode": Value Change {
            n89 = event-data() -> ("NewVal"=w150:bool)  [unwired: 1 in, 5 out]
            n90 = case shown="True" w150 {
              frame False {
              }
              frame True {
                n91 = property on="exposure::4" class="DigNum (strict)"("Val(Sgnl)"=500.0) -> ()  [unwired: 2 in, 2 out]
                n92 = property on="exposure::5" class="DigNum (strict)"("Val(Sgnl)"=0.001) -> ()  [unwired: 2 in, 2 out]
                n93 = property on="exposure::2" class="DigNum (strict)"("Val(Sgnl)"=0.002) -> ()  [unwired: 2 in, 2 out]
                n94 = property on="exposure::3" class="DigNum (strict)"("Val(Sgnl)"=0.001) -> ()  [unwired: 2 in, 2 out]
                n95 = property on="exposure::6" class="DigNum (strict)"("Val(Sgnl)"=0.001) -> ()  [unwired: 2 in, 2 out]
                n96 = property on="exposure::9" class="DigNum (strict)"("Val(Sgnl)"=0.001) -> ()  [unwired: 2 in, 2 out]
                n97 = property on="exposure::7" class="DigNum (strict)"("Val(Sgnl)"=0.001) -> ()  [unwired: 2 in, 2 out]
                n98 = property on="exposure::8" class="DigNum (strict)"("Val(Sgnl)"=0.001) -> ()  [unwired: 2 in, 2 out]
                n99 = property on="exposure::10" class="DigNum (strict)"("Val(Sgnl)"=1000.0) -> ()  [unwired: 2 in, 2 out]
              }
            }
            n100 = Bundle By Name(cluster=w152, "kHzMode"=w150) -> (w151:T32)
          }
          event "GUIdevice 1": Value Change {
            n101 = event-data() -> ("NewVal"=w164:string)  [unwired: 1 in, 5 out]
            n102 = local write "GUIdevice 1"(w164) -> ()
            n103 = flat-sequence {
              tunnel: [w173] -> w168
              tunnel: w169 -> [w172]
              tunnel: w164 -> [w171]
              frame #0 {
                # "Set FP title as device name"
                n104 = control-ref of="This VI"() -> (w176:refnum<vi>)
                n105 = Concatenate Strings(w171, "_GUI ") -> (w175:string)
                n106 = property class="VI"(reference=w176, error in=w172, "Front Panel.Title"=w175) -> (error out=w173:errorcluster)  [unwired: 1 out]
              }
            }
            n107 = call <vilib>:"Add State(s) to Queue__jki_lib_state_machine.vi"("State(s) in Front (\"\")"="UI: Stop SuperGUI\nUI: Start SuperGUI", "State(s) in (\"\")"=w167) -> ("States Out"=w166:string)  [unwired: 13 in]
          }
          event "Select device": Value Change {
            n108 = event-data() -> ()  [unwired: 1 in, 6 out]
            n109 = local write "GUIdevice 1"("Select device") -> ()
            n110 = flat-sequence {
              tunnel: [w186] -> w181
              tunnel: w182 -> [w185]
              tunnel: "Select device" -> [w184]
              frame #0 {
                # "Set FP title as device name"
                n111 = control-ref of="This VI"() -> (w189:refnum<vi>)
                n112 = Concatenate Strings(w184, "_GUI ") -> (w188:string)
                n113 = property class="VI"(reference=w189, error in=w185, "Front Panel.Title"=w188) -> (error out=w186:errorcluster)  [unwired: 1 out]
              }
            }
            n114 = call <vilib>:"Add State(s) to Queue__jki_lib_state_machine.vi"("State(s) in Front (\"\")"="UI: Stop SuperGUI\nUI: Start SuperGUI", "State(s) in (\"\")"=w179) -> ("States Out"=w178:string)  [unwired: 13 in]
          }
          event "Refresh Button": Value Change {
            n115 = event-data() -> ()  [unwired: 1 in, 6 out]
            n116 = call <vilib>:"Add State(s) to Queue__jki_lib_state_machine.vi"("State(s) in Front (\"\")"="UI: Stop SuperGUI\nUI: Start SuperGUI", "State(s) in (\"\")"=w192) -> ("States Out"=w191:string)  [unwired: 13 in]
          }
          event Panel Close? {
            # "Discard the event because we'll close the front panel ourselves in Macro: Exit"
            # "Close Panel button (pressed) Event\n(this executes Macro: Exit to terminate the VI)"
            n117 = event-data() -> ()  [unwired: 1 in, 1 out]
            n118 = event-data("Discard?"=TRUE) -> ()  [unwired: 1 in, 1 out]
            n119 = call <vilib>:"Add State(s) to Queue__jki_lib_state_machine.vi"("State(s) in Front (\"\")"="Macro: Exit", "State(s) in (\"\")"=w200) -> ("States Out"=w199:string)  [unwired: 13 in]
          }
        }
      }
      frame "---------- Core ----------" {
        # "Do not put any code in this frame.\n(it is a separator no-op)"
        n120 = call <vilib>:"Add State(s) to Queue__jki_lib_state_machine.vi"("State(s) in (\"\")"=w204) -> ("States Out"=w203:string)  [unwired: 14 in]
      }
      frame Default {
        w214 = 42 items=["No error", "Argument error", "Memory is full", "Out of zone", "End of file", "File already open", "Generic file I/O error", "File not found", "File permission error", "Disk is full", "Duplicate path", "Too many files open", "System feature not enabled", "Resource file not found", "Cannot add resource", "Resource not found", "Image not found", "Image memory error", "Pen does not exist", "Config type invalid", "Config token not found", "Config parse error", "Config memory error", "Bad external code format", "Bad external code offset", "External code not present", "Null window", "Destroy window error", "Null menu", "Print aborted", "Bad print record", "Print driver error", "Windows error during printing", "Memory error during printing", "Print dialog error", "Generic print error", "Invalid device refnum", "Device not found", "Device parameter error", "Device unit error", "Cannot open device", "Device call aborted", "Generic error", "Cancelled by user", "Object ID too low", "Object ID too high", "Object not in heap", "Unknown heap", "Unknown object (invalid DefProc)", "Unknown object (DefProc not in table)", "Message out of range", "Invalid (null) method", "Unknown message", "Manager call not supported", "Bad address", "Network operation in progress", "Network operation timed out", "Connection is busy", "Network attribute not supported", "Network error", "Address in use", "System out of memory", "Connection aborted", "Connection refused", "Not connected", "Already connected", "Connection closed", "Initialization error (interapplication manager)", "Bad occurrence", "Wait on unbound occurrence handler", "Occurrence queue overflow", "Datalog type conflict", "Unused", "Unrecognized type (interapplication manager)", "Memory corrupt", "Failed to make temporary DLL", "Old CIN version", "Drag socket not found", "Failed to load drop-object", "Failed to register OLE object", "Failed to release OLE object", "Format specifier type mismatch", "Unknown format specifier", "Too few format specifiers", "Too many format specifiers", "Scan failed", "Newer CIN version", "Error converting to variant", "Runtime menu error", "Password tampered", "Variant attribute not found", "Incompatible variant data type", "Event data is not available", "Event Store is not present", "Occurrence is not found", "Event Queue is not created", "Event info is not available", "Refnum passed is NULL", "Error retrieving Class GUID", "Error retrieving CoClass GUID", "Error retrieving TypeLib GUID.", "Bad built application magic bytes.", "Specific driver is different from the specific driver associated with the Logical Name.", "There is no session opened to the class driver.", "Max Error", "MAX - Error with config objects", "MAX - Error loading configuration", "MAX - Group not supported"]
        # "Current State"
        # "Do not delete, rename, or modify this frame.\n(this is used to capture unhandled states and typos)"
        # "Handle mistyped state name (developer tool)"
        n121 = Format Into String(format string="Software Exception: Unhandled State \"%s\"." ("message"), error in=w210, w205) -> (resulting string=w213:string, error out=w212:errorcluster)  [unwired: 1 in]
        n122 = call <vilib>:"Error Cluster From Error Code.vi"("show call chain? (False)"=TRUE, "error in (no error)"=w212, "error message (\"\")"=w213, "error code (0)"=w214) -> ("error out"=w211:errorcluster)  [unwired: 5 in]
        n123 = call <vilib>:"Add State(s) to Queue__jki_lib_state_machine.vi"("State(s) in (\"\")"=w209) -> ("States Out"=w208:string)  [unwired: 14 in]
      }
      frame "Initialize Core Data" {
        # "Do not delete, rename, or modify this frame.\n(this is used to determine panel behavior on exit)"
        # "originally closed?"
        # "exe?"
        # "If panel starts closed or is an EXE, then close it when we exit"
        n124 = property class="VI"() -> ("Front Panel.Open"=w223:bool)  [unwired: 2 in, 2 out]
        n125 = property class="App"() -> ("App.Kind"=w222:T29)  [unwired: 2 in, 2 out]
        n126 = control-ref of="Current VI Reference"() -> (w216:refnum<vi>)
        n127 = Not(x=w223) -> (.not. x?=w220:bool)
        n128 = Equal?(x=w222, y=T29."Run Time System" ("Application:Kind")) -> (x = y?=w219:bool)
        n129 = Or(x=w220, y=w219) -> (x .or. y?=w217:bool)
        n130 = Bundle By Name(cluster=w218, "Core.Current VI Reference"=w216, "Core.Close Panel on Exit?"=w217) -> (w225:T32)
        n131 = call <vilib>:"Add State(s) to Queue__jki_lib_state_machine.vi"("State(s) in (\"\")"=w227) -> ("States Out"=w226:string)  [unwired: 14 in]
      }
      frame "Error Handler" {
        # "Unhandled Error -- Display it"
        # "Handle any errors here.\nYou can also output any states to clean-up after errors occur"
        # "Clear error"
        n132 = call <vilib>:"General Error Handler.vi"("error in (no error)"=w229) -> ()  [unwired: 10 in, 5 out]
        n133 = call <vilib>:"Add State(s) to Queue__jki_lib_state_machine.vi"("State(s) in Front (\"\")"="/* Post Error States", "State(s) in (\"\")"=w233) -> ("States Out"=w232:string)  [unwired: 13 in]
      }
      frame "Exit" {
        # "Do not put any code in this frame.\n(No errors that occur here will be handled.)"
        n134 = call <vilib>:"Add State(s) to Queue__jki_lib_state_machine.vi"("State(s) in (\"\")"=w238) -> ("States Out"=w237:string)  [unwired: 14 in]
      }
      frame "---------- Data ----------" {
        # "Do not put any code in this frame.\n(It is a separator no-op. You can make a copy of this frame to create a new Data frame)"
        n135 = call <vilib>:"Add State(s) to Queue__jki_lib_state_machine.vi"("State(s) in (\"\")"=w242) -> ("States Out"=w241:string)  [unwired: 14 in]
      }
      frame "Data: Initialize" {
        w243 = TRUE  # kHzMode
        w244 = T33 {"STOP queue"=refnum, "SuperGUI ref"=refnum}  # SuperGUI
        w245 = T34 {"Current VI Reference"=refnum, "Close Panel on Exit?"=FALSE}  # Core
        w247 = TRUE  # DiodeMode
        # "Initialize the shift-register data, here.\n(data names are defined by what you wire into the bundle function)"
        n136 = Bundle("Core"=w245, "DiodeMode"=w247, "active cams"="active cams", "SuperGUI"=w244, "kHzMode"=w243) -> (w249:T32)  [unwired: 1 in]
        n137 = call <vilib>:"Add State(s) to Queue__jki_lib_state_machine.vi"("State(s) in (\"\")"=w251) -> ("States Out"=w250:string)  [unwired: 14 in]
      }
      frame "Data: Cleanup" {
        # "Cleanup any data and references, here.\n(this is called automatically, by the Macro: Exit)"
        n138 = Unbundle By Name(w252) -> ("Core.Current VI Reference"=w255:refnum<vi>)
        n139 = Close Reference(reference=w255, error in (no error)=w254) -> (error out=w253:errorcluster)
        n140 = call <vilib>:"Add State(s) to Queue__jki_lib_state_machine.vi"("State(s) in (\"\")"=w257) -> ("States Out"=w256:string)  [unwired: 14 in]
      }
      frame "---------- UI ----------" {
        # "Do not put any code in this frame.\n(It is a separator no-op. You can make a copy of this frame to create a new UI frame)"
        n141 = call <vilib>:"Add State(s) to Queue__jki_lib_state_machine.vi"("State(s) in (\"\")"=w261) -> ("States Out"=w260:string)  [unwired: 14 in]
      }
      frame "UI: Initialize" {
        # "Initialize the User Interface, here.\n(this is called automatically, by the Macro: Init)"
        n142 = for {
          tunnel: string[] ["Point Grey Camera", "Manta Camera", "Photometrics Cam", "Basler Camera"] -> [w270] mode=indexing
          tunnel: [w269] -> w262 mode=concatenating
          n143 = call "getDevices.vi"("Device Class"=w270) -> ("All Devices"=w269:string[])
        }
        n144 = call <userlib>:"Fit VI window to Largest Dec__ogtk.vi"("error in (no error)"=w265) -> ("error out"=w264:errorcluster)  [unwired: 5 in, 1 out]
        n145 = property on="Select device" class="CmbBox"("Strings[]"=w262) -> ()  [unwired: 2 in, 2 out]
        n146 = call <vilib>:"Add State(s) to Queue__jki_lib_state_machine.vi"("State(s) in (\"\")"=w268) -> ("States Out"=w267:string)  [unwired: 14 in]
      }
      frame "UI: Get Device Name" {
        # "Initialize the User Interface, here.\n(this is called automatically, by the Macro: Init)"
        n147 = First Call?() -> (First Call?: T/F=w273:bool)
        n148 = case shown="True" w273 {
          tunnel: w272 -> [w277 w279]
          tunnel: [w277 w278] -> w271
          frame False {
          }
          frame True {
            n149 = disable-structure "Get Device name from control for vi mode\nand command line arg for exe" shown="RUN_TIME_ENGINE==True" {
              disable-tunnel: w279 -> [w280 w282]
              disable-tunnel: [w280 w281] -> w278
              frame condition #0 (active) {
              }
              frame condition #1 {
                n150 = control-ref of="This Application"() -> (w290:refnum<vi>)
                n151 = property class="App"(reference=w290) -> ("App.Args"=w289:string[])  [unwired: 1 in, 2 out]
                n152 = Index Array(array=w289, index #1=1 ("index")) -> (element #1=w283:string)  [unwired: 2 in, 2 out]
                n153 = Empty String/Path?(string/path=w283) -> (empty?=w287:bool)
                n154 = control-ref of="This VI"() -> (w286:refnum<vi>)
                n155 = case shown="False" w287 {
                  tunnel: w283 -> [w291 _]
                  frame False {
                    n156 = local write "GUIdevice 1"(w291) -> ()
                  }
                  frame True {
                  }
                }
                n157 = Concatenate Strings(w283, "_GUI ") -> (w285:string)
                n158 = property class="VI"(reference=w286, error in=w282, "Front Panel.Title"=w285) -> (error out=w281:errorcluster)  [unwired: 1 out]
              }
            }
          }
        }
        n159 = call <vilib>:"Add State(s) to Queue__jki_lib_state_machine.vi"("State(s) in (\"\")"=w276) -> ("States Out"=w275:string)  [unwired: 14 in]
      }
      frame "UI: Start SuperGUI" {
        # "create stop queue for supergui and its clones"
        # "x100 abort will be dependent on caller VI\nx80 abort will be independent of caller vi, this will abort vi when labview is closed."
        # "Start SuperGUI asynchronous way"
        n160 = vi-ref "GUI_Master_subvi_reentrant_queues.vi"() -> (w294:refnum<vi>)
        n161 = property class="VI"(reference=w294) -> ("Path"=w293:path)  [unwired: 1 in, 2 out]
        n162 = Create User Event(user event datatype=T30 {"EventEnum"=enum."new data", "Device name"="Device name"} ("New Event"), error in=w296) -> (user event=w297:refnum<user-event>, error out=w303:errorcluster)
        "tcp data event" <- w297
        n163 = control-ref of="This Application"() -> (w300:refnum<vi>)
        n164 = control-ref of="This VI"() -> (w299:refnum<vi>)
        n165 = Open VI Reference(type specifier VI Refnum (for type only)=refnum<vi> refnum, vi path=w293, options=256) -> (vi reference=w309:refnum<vi>, error out=w308:errorcluster)  [unwired: 3 in]
        n166 = register-events(w297) -> ()  [unwired: 2 in, 2 out]
        n167 = call "supergui create stop queue.vi"() -> ("STOP Queue out"=w305:refnum<queue>)  [unwired: 11 in]
        n168 = Current VI's Menubar() -> (w298:refnum<k9>)
        n169 = call-by-ref "Start Asynchronous Call"(reference=w309, error in=w308, "STOP Queue in"=w305, "This Application"=w300, 8:"error in (no error)"=w303, "tcp data event"=w297, "Caller menu reference"=w298, "Caller VI ref"=w299) -> (reference out=w292:refnum<vi>, error out=w295:errorcluster)  [unwired: 5 in, 1 out]
        n170 = Bundle By Name(cluster=w302, "SuperGUI.SuperGUI ref"=w292, "SuperGUI.STOP queue"=w305) -> (w301:T32)
        n171 = call <vilib>:"Add State(s) to Queue__jki_lib_state_machine.vi"("State(s) in (\"\")"=w311) -> ("States Out"=w310:string)  [unwired: 14 in]
      }
      frame "UI: Stop SuperGUI" {
        # "Stop Supergui Clone and wait until it exit properly"
        n172 = Unbundle By Name(w314) -> ("SuperGUI.SuperGUI ref"=w316:refnum<vi>, "SuperGUI.STOP queue"=w315:refnum<queue>)
        n173 = Release Queue(queue=w315, error in (no error)=w313) -> (error out=w317:errorcluster)  [unwired: 1 in, 2 out]
        n174 = call-by-ref "Wait On Asynchronous Call"(reference=w316, error in=w317) -> ("error out"=w312:errorcluster)  [unwired: 11 in, 2 out]
        n175 = call <vilib>:"Add State(s) to Queue__jki_lib_state_machine.vi"("State(s) in (\"\")"=w319) -> ("States Out"=w318:string)  [unwired: 14 in]
      }
      frame "UI: Cursor Set" {
        # "Argument"
        # "Set and Unset Cursor Busy.\n(Usage: \"UI: Cursor Set >> Busy|Idle\")"
        n176 = case shown="\"Idle\", Default" w320 {
          tunnel: w322 -> [w327 w329]
          tunnel: [w326 w328] -> w321
          frame "Idle", Default {
            n177 = call <vilib>:"Unset Busy.vi"("error in (no error)"=w327) -> ("error out"=w326:errorcluster)  [unwired: 10 in]
          }
          frame "Busy" {
            n178 = call <vilib>:"Set Busy.vi"("error in (no error)"=w329) -> ("error out"=w328:errorcluster)  [unwired: 9 in, 1 out]
          }
        }
        n179 = call <vilib>:"Add State(s) to Queue__jki_lib_state_machine.vi"("State(s) in (\"\")"=w325) -> ("States Out"=w324:string)  [unwired: 14 in]
      }
      frame "UI: Front Panel State" {
        # "Argument"
        # "Set Front Panel Open or Closed\n(Usage: \"UI: Front Panel State >> Open|Close\")"
        n180 = Unbundle By Name(w332) -> ("Core.Current VI Reference"=w331:refnum<vi>)
        n181 = case shown="\"Open\", Default" w330 {
          tunnel: w334 -> [w340 w353]
          tunnel: [w342 w354] -> w333
          tunnel: w331 -> [w341 w351]
          frame "Open", Default {
            n182 = property class="VI"(reference=w341, error in=w340) -> (reference out=w338:refnum<vi>, error out=w339:errorcluster, "Front Panel.Open"=w337:bool)
            n183 = case shown="False" w337 {
              tunnel: [w345 w348] -> w342
              tunnel: w339 -> [w344 w348]
              tunnel: w338 -> [w343 _]
              frame False {
                n184 = invoke class="VI" method="FP.Open"(reference=w343, error in=w344, "Activate"=TRUE, "State"=T31."Standard") -> (error out=w345:errorcluster)  [unwired: 1 in, 4 out]
              }
              frame True {
              }
            }
          }
          frame "Close" {
            n185 = property class="VI"(reference=w351, error in=w353) -> (reference out=w350:refnum<vi>, error out=w352:errorcluster, "Front Panel.Open"=w349:bool)
            n186 = case shown="True" w349 {
              tunnel: [w355 w358] -> w354
              tunnel: w352 -> [w355 w357]
              tunnel: w350 -> [_ w356]
              frame False {
              }
              frame True {
                n187 = invoke class="VI" method="FP.Close"(reference=w356, error in=w357) -> (error out=w358:errorcluster)  [unwired: 1 in, 2 out]
              }
            }
          }
        }
        n188 = call <vilib>:"Add State(s) to Queue__jki_lib_state_machine.vi"("State(s) in (\"\")"=w336) -> ("States Out"=w335:string)  [unwired: 14 in]
      }
      frame "---------- Macro ----------" {
        # "Do not put any code in this frame.\n(It is a separator no-op. You can make a copy of this frame to create a new Macro frame)"
        n189 = call <vilib>:"Add State(s) to Queue__jki_lib_state_machine.vi"("State(s) in (\"\")"=w362) -> ("States Out"=w361:string)  [unwired: 14 in]
      }
      frame "Macro: Initialize" {
        # "Initialization Macro\n(This is called once, when the VI starts)"
        n190 = call <vilib>:"Add State(s) to Queue__jki_lib_state_machine.vi"("State(s) in Front (\"\")"="Data: Initialize\nInitialize Core Data\nUI: Initialize\nUI: Get Device Name\nUI: Start SuperGUI\nUI: Front Panel State >> Open", "State(s) in (\"\")"=w367) -> ("States Out"=w366:string)  [unwired: 13 in]
      }
      frame "Macro: Exit" {
        # "Exit Macro\n(This is called once, when the VI exits)"
        n191 = Unbundle By Name(w374) -> ("Core.Close Panel on Exit?"=w373:bool)
        n192 = Select(t="UI: Front Panel State >> Close", s=w373, f="") -> (s? t:f=w370:string)
        n193 = call <vilib>:"Add State(s) to Queue__jki_lib_state_machine.vi"("State(s) in (\"\")"=w370, "State(s) at Back (\"\")"="Data: Cleanup\nExit") -> ("States Out"=w368:string)  [unwired: 13 in]
        n194 = call <vilib>:"Add State(s) to Queue__jki_lib_state_machine.vi"("State(s) in Front (\"\")"=w368, "State(s) in (\"\")"=w377) -> ("States Out"=w376:string)  [unwired: 13 in]
      }
      frame "---------- New Category ----------" {
        # "Template Separator\n(You can make a copy of, or modify, this frame)"
        n195 = call <vilib>:"Add State(s) to Queue__jki_lib_state_machine.vi"("State(s) in (\"\")"=w381) -> ("States Out"=w380:string)  [unwired: 14 in]
      }
      frame "New Category: 1" {
        # "Your code here.\n(You can make a copy of, or modify, this frame)"
        n196 = call <vilib>:"Add State(s) to Queue__jki_lib_state_machine.vi"("State(s) in (\"\")"=w385) -> ("States Out"=w384:string)  [unwired: 14 in]
      }
      frame "New Category: 2" {
        # "Your code here.\n(You can make a copy of, or modify, this frame)"
        n197 = call <vilib>:"Add State(s) to Queue__jki_lib_state_machine.vi"("State(s) in (\"\")"=w389) -> ("States Out"=w388:string)  [unwired: 14 in]
      }
    }
    n198 = for {
      tunnel: w84 -> [w111]
      tunnel: w83 -> [w115]
      tunnel: w81 -> [w112] mode=indexing
      tunnel: w80 -> [w108]
      (unwired) u32 16774656 ("Color")
      n199 = call-poly <userlib>:"Filter 1D Array__ogtk.vi"("items to filter"=w112, "array"=w115) -> ("filtered item indices"=w116:i32[])  [unwired: 4 in, 1 out]
      n200 = Index Array(array=w116) -> (element=w110:i32)  [unwired: 1 in]
      n201 = Index Array(array=w108, index=w110) -> (element=w109:T23)
      n202 = Unbundle By Name(w109) -> ("TargetSize.Y::10"=w107:refnum<vi>, "TargetSize.X::10"=w106:refnum<vi>)
      n203 = Index Array(array=w111, index=w110) -> (element=w114:T8)
      n204 = property class="DigNum (strict)"(reference=w107) -> ("Value"=w105:dbl)  [unwired: 1 in, 2 out]
      n205 = property class="DigNum (strict)"(reference=w106) -> ("Value"=w104:dbl)  [unwired: 1 in, 2 out]
      n206 = Unbundle By Name(w114) -> ("Target.X::10"=w118:refnum<vi>, "Target.Y::10"=w117:refnum<vi>)
      n207 = property class="DigNum (strict)"(reference=w118) -> ("Value"=w100:dbl)  [unwired: 1 in, 2 out]
      n208 = property class="DigNum (strict)"(reference=w117) -> ("Value"=w99:dbl)  [unwired: 1 in, 2 out]
      n209 = Bundle("Value"=w100, "Value"=w99) -> (w98:cluster{"Value":dbl, "Value":dbl})  [unwired: 1 in]
      n210 = Bundle("Value"=w105, "Value"=w104) -> (w97:cluster{"Value":dbl, "Value":dbl})  [unwired: 1 in]
      n211 = Bundle By Name(cluster=T27 {"Draw"=TRUE, "Target"={"x"=20.0, "y"=20.0}, "Size"={"x"=20.0, "y"=20.0}, "Angle"=1250067.0, "Color"=1250067, "Thickness"=3, "CrosshairLabel"=""} ("Crosshair"), "Draw"=TRUE, "Target"=w98, "Size"=w97, "Angle"=0.0, "Color"="Color Box") -> (w102:T27)
      n212 = call "draw crosshair imaq.vi"("Crosshair"=w102, "Bounding Rectangle"=T28 {"Left"=0, "Top"=0, "Right"=0, "Bottom"=0}, "image in"=w112) -> ("error out"=→"error out":errorcluster)  [unwired: 7 in, 1 out]
    }
  }
